vi "MT Rayleigh Selective Fading profile (Gans).vi"(0 "profile length (samples)":i32=1000, 1 "number of paths":i32=1, 5 "sampling frequency (Hz)":dbl=1.0 format="%.2f", 7 "doppler spread (Hz)":dbl=0.01 format="%.2p", 9 "seed in (0xFFFFFFFF)":i32=-1 format="%.0x", 11 "error in (no error)":errorcluster, 12 "fading variance":dbl=1.0 format="%.2f", 13 "reset? (T)":bool=TRUE) -> (4 "fading profile":cdb[][](array[numeric]), 10 "seed out":i32 format="%.0x", 15 "error out":errorcluster)   [LabVIEW 2020, in "niDMT.lvlib"]
doc: "This polymorphic instance generates a Rayleigh selective-fading profile for the multipath channel. The envelope for each path statistically obeys the Rayleigh distribution implemented using the Gans fading model."
uses:
  <vilib>/addons/Modulation/niDMT.lvlib
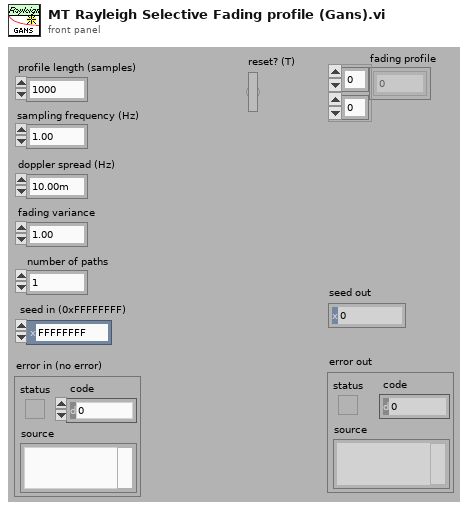
[diagram p1: front panel]
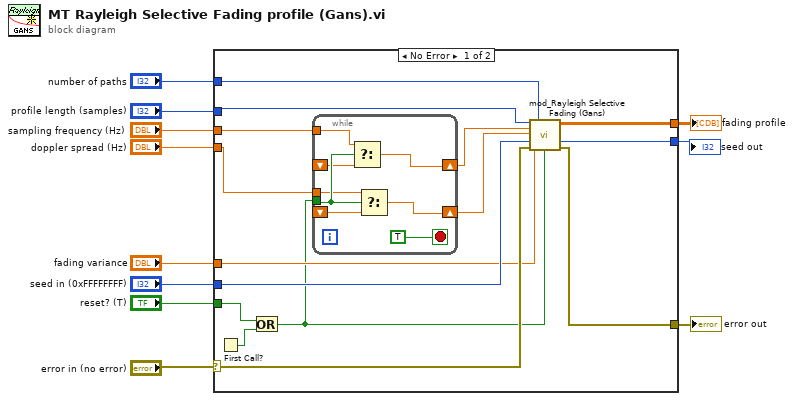
[diagram p0: block diagram]
diagram:
  n1 = case shown="No Error" "error in (no error)" {
    selector: "error in (no error)" -> [w17 w35]
    tunnel: "profile length (samples)" -> [w21 _]
    tunnel: [w13 _] -> w2
    tunnel: [w12 w35] -> w10
    tunnel: "sampling frequency (Hz)" -> [w24 _]
    tunnel: "doppler spread (Hz)" -> [w23 _]
    tunnel: "fading variance" -> [w16 _]
    tunnel: "reset? (T)" -> [w25 _]
    tunnel: "seed in (0xFFFFFFFF)" -> [w18 _]
    tunnel: [w14 _] -> w3
    tunnel: "number of paths" -> [w22 _]
    frame No Error {
      n2 = First Call?() -> (First Call?: T/F=w26:bool)
      n3 = Or(x=w25, y=w26) -> (x .or. y?=w15:bool)
      n4 = while {
        tunnel: w15 -> [w33]
        tunnel: w24 -> [w32]
        shift-right: [w31] -> w20
        shift-left: _ -> [w30]
        tunnel: w23 -> [w29]
        shift-right: [w28] -> w19
        shift-left: _ -> [w27]
        stop <- TRUE stop-if-true
        n5 = Select(t=w32, s=w33, f=w30) -> (s? t:f=w31:dbl)
        n6 = Select(t=w29, s=w33, f=w27) -> (s? t:f=w28:dbl)
      }
      n7 = call <vilib>:"mod_Rayleigh Selective Fading (Gans).vi"("profile length (samples)"=w21, "number of paths"=w22, "sampling frequency (Hz)"=w20, "doppler spread (Hz)"=w19, "seed in (0xFFFFFFFF)"=w18, "error in (no error)"=w17, "fading variance"=w16, "reset? (T)"=w15) -> ("Rayleigh fading profile"=w13:cdb[][], "seed out"=w14:i32, "error out"=w12:errorcluster)  [unwired: 5 out]
    }
    frame Error {
    }
  }
  "error out" <- w10
  "seed out" <- w3
  "fading profile" <- w2
